vi "Process.vi"(8 "error in":errorcluster, 11 "UI.Lockin.Main":refnum<class "UI.Lockin.lvclass">) -> (0 "error out":errorcluster, 3 "UI.Lockin.Main out":refnum<class "UI.Lockin.lvclass">)   [LabVIEW 2019, in "UI.Lockin.lvclass"]
doc: "---------------------------------------------------------------\nJKI State Machine Objects™\nhttp://jki.net/state-machine-objects/\nCopyright (C) 2005-2015, JKI <info@jki.net>\nALL RIGHTS RESERVED"
uses:
  UI.Lockin.lvclass
  C:/Program Files (x86)/National Instruments/LabVIEW 2019/vi.lib/JKI/JKI SMO/SMO/SMO.lvclass
  <vilib>/JKI/JKI SMO/SMO/SMO.lvclass/SMO.ctl
  <vilib>/JKI/JKI SMO/SMO/Private/ReftoDVR--SMO.vi
  <userlib>/LevyLab/Instrument Framework/SMOs/Instrument UI/Instrument UI.lvclass
  C:/Program Files (x86)/National Instruments/LabVIEW 2019/vi.lib/JKI/JKI SMO/SMO.UI/SMO.UI.lvclass
  <vilib>/JKI/JKI SMO/SMO/SMO.lvclass
  <vilib>/JKI/JKI SMO/SMO.UI/SMO.UI.lvclass
panel:
  in  "configGenerator":bool
  in  "Shutdown":bool
  in  "configDSP":bool
  in  "configDAQ":bool
  in  "show Scope":bool
  # "For instructions on how to use the JKI State Machine Objects, examples and video tutorials, visit:\nhttp://jki.net/state-machine-objects/\n\nJKI State Machine Objects™\nhttp://jki.net/state-machine-objects/\nCopyright (C) 2005-2015, JKI <info@jki.net>\nALL RIGHTS RESERVED"
  # "mainUI"
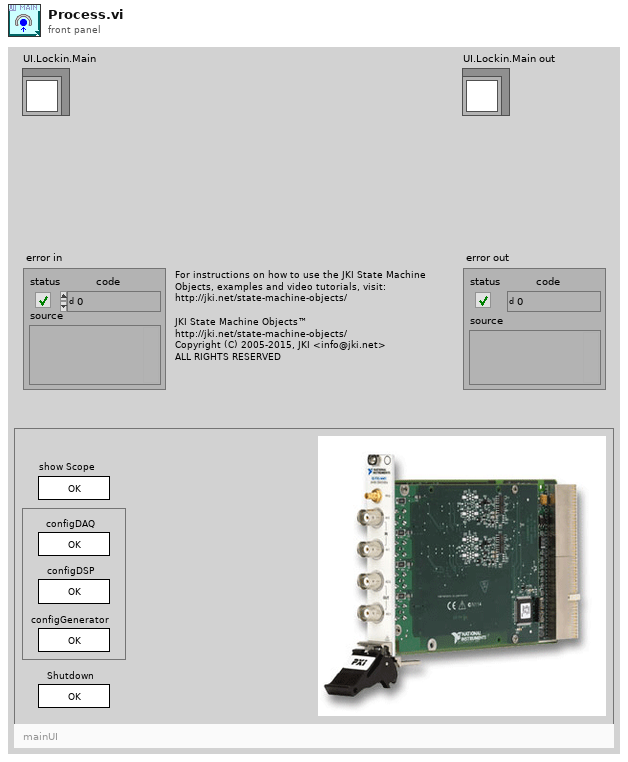
[diagram p1: front panel]
types:
  T1 = enum32{"invalid app kind", "Development System", "Run Time System", "Student Edition", "Embedded LabVIEW", "Evaluation", "Custom"}
  T2 = enum32{"Invalid", "Standard", "Closed", "Hidden", "Minimized", "Maximized"}
  T3 = enum32{"Bad", "Idle", "Run top level", "Running"}
  T4 = cluster{"Core":cluster{"Current VI Reference":refnum<vi>, "Close Panel on Exit?":bool, "error":errorcluster}, "SelfRef":refnum<class "UI.Lockin.lvclass">}
  T5 = cluster{"Current VI Reference":refnum<vi>, "Close Panel on Exit?":bool, "error":errorcluster}
  T6 = typedef "SMO.lvclass/Protected Events.ctl" = cluster{"StopProcesses":refnum<user-event>, "AbortProcesses":refnum<user-event>, "Config Changed":refnum<user-event>, "Dependency":refnum<user-event>}
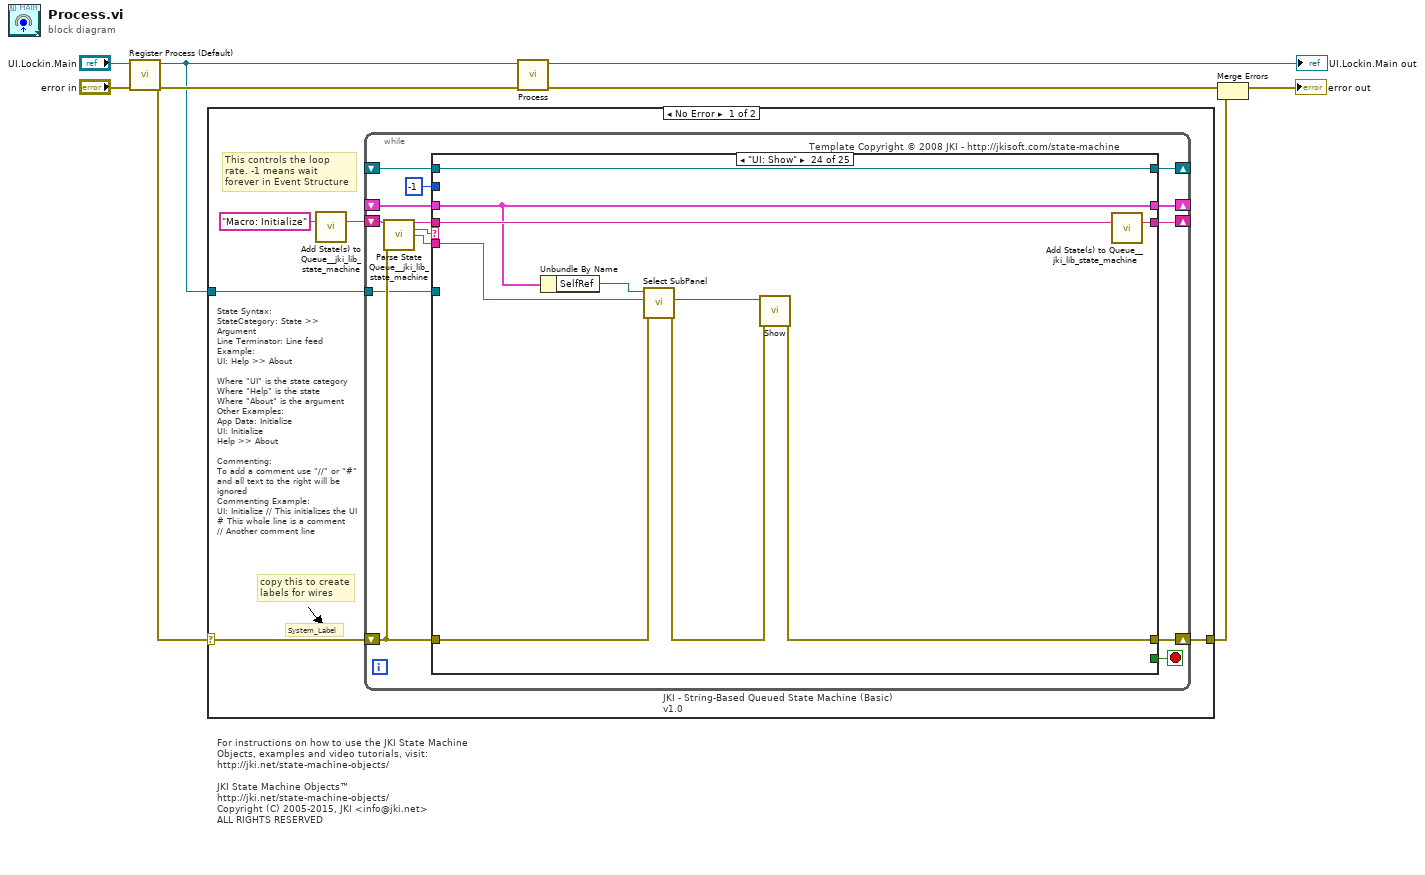
[diagram p0: block diagram]
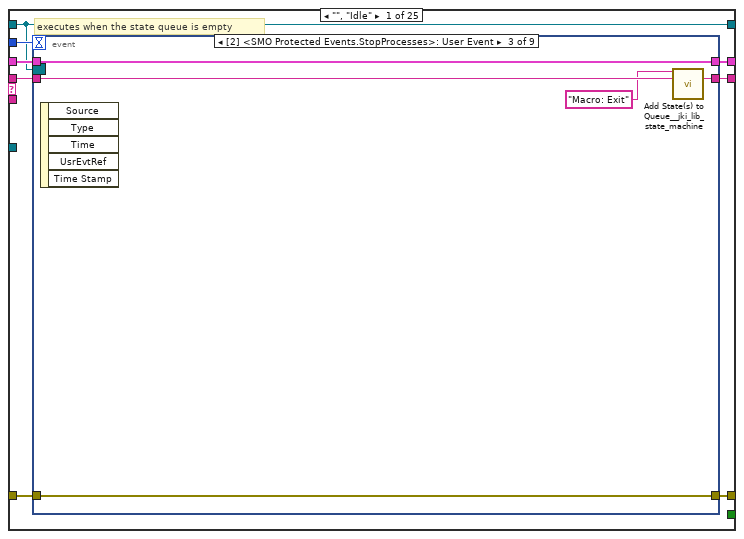
[diagram p2: hidden frame]
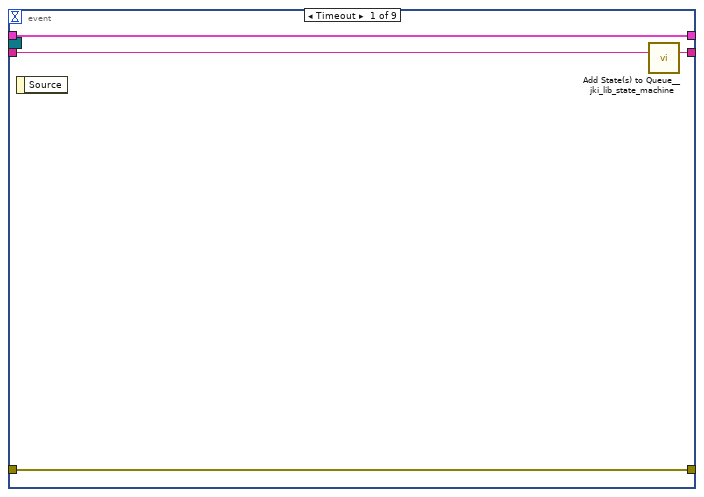
[diagram p3: hidden frame]
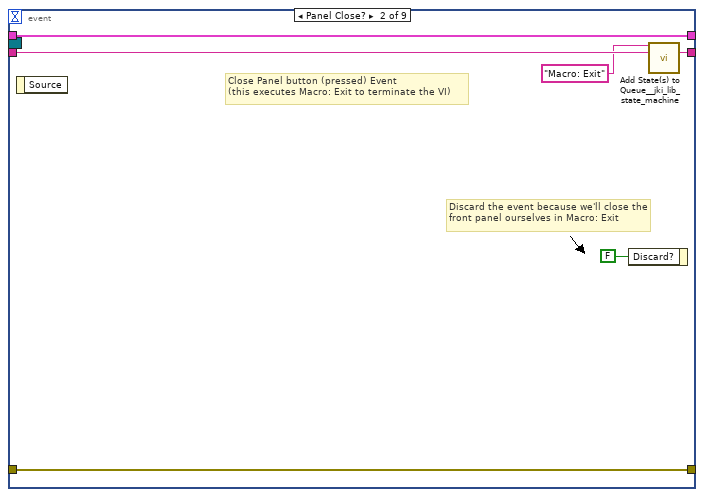
[diagram p4: hidden frame]
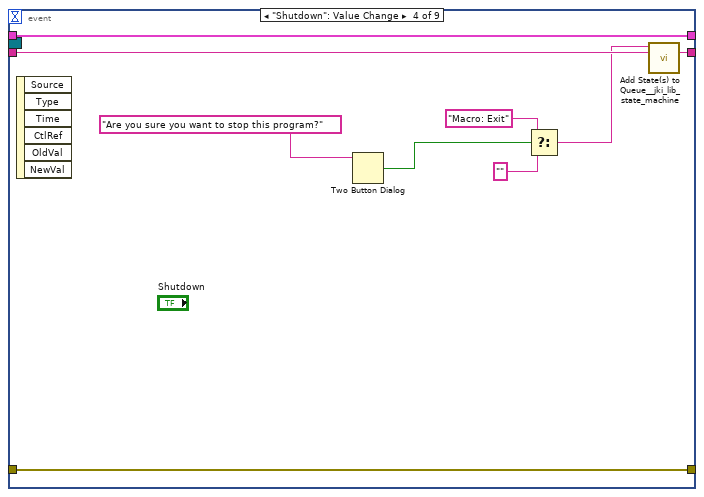
[diagram p5: hidden frame]
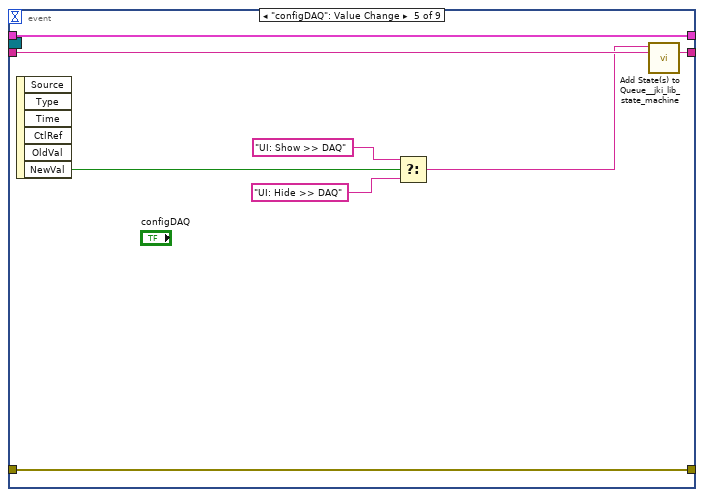
[diagram p6: hidden frame]
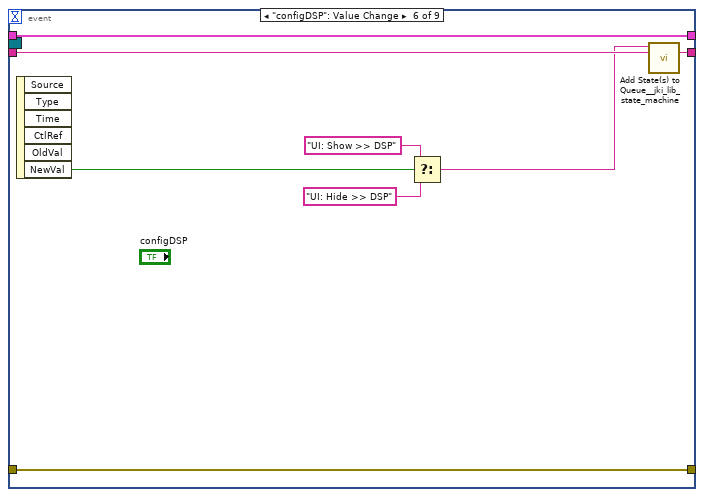
[diagram p7: hidden frame]
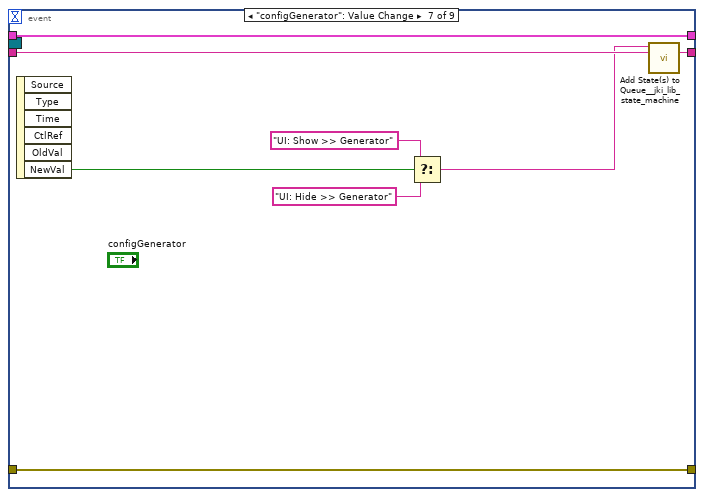
[diagram p8: hidden frame]
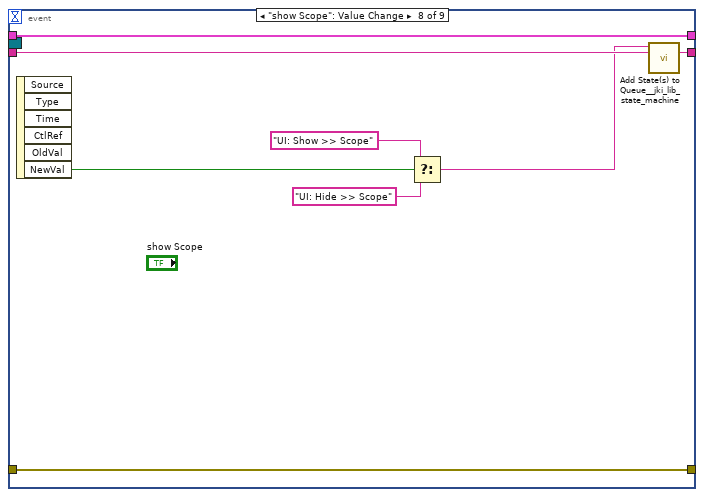
[diagram p9: hidden frame]
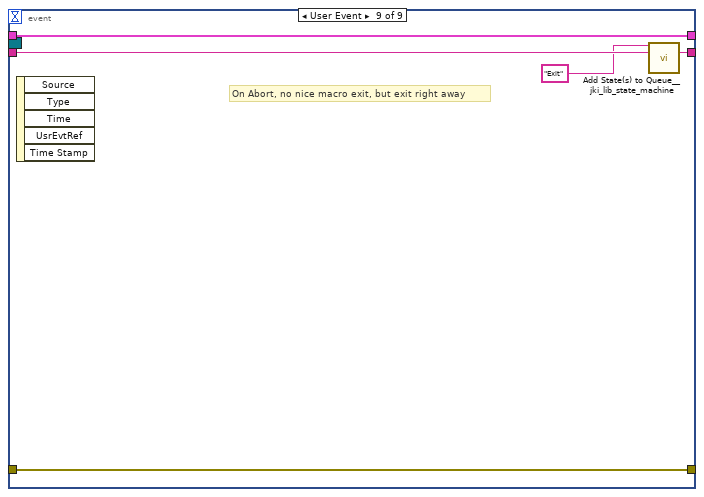
[diagram p10: hidden frame]
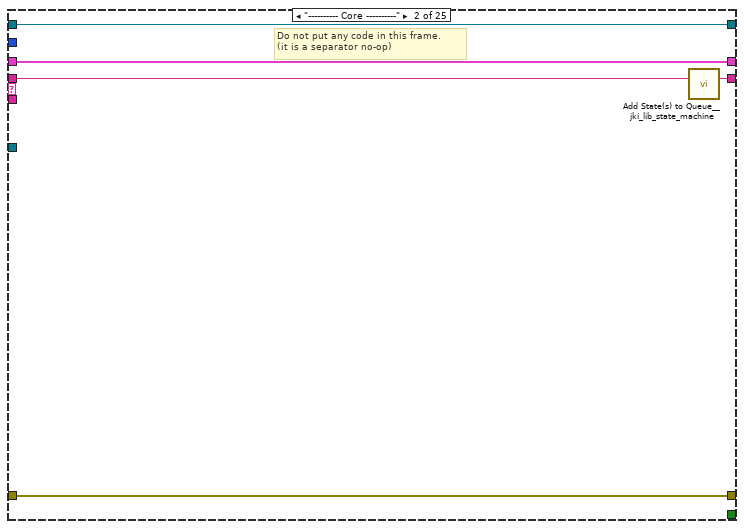
[diagram p11: hidden frame]
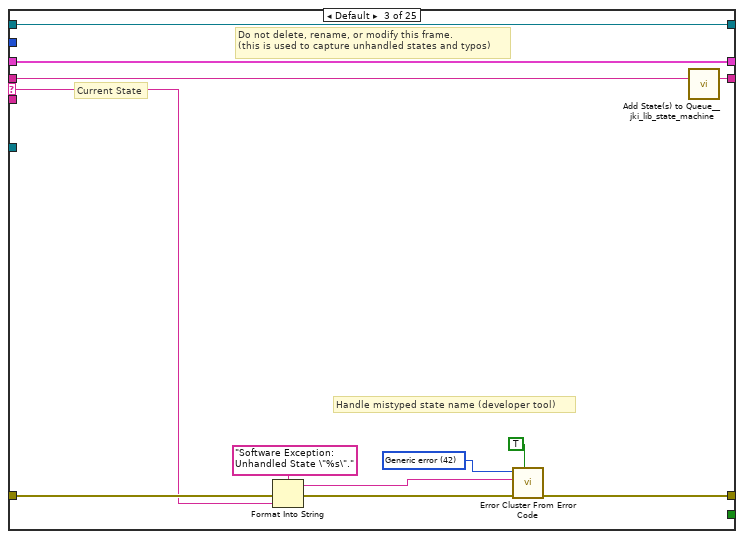
[diagram p12: hidden frame]
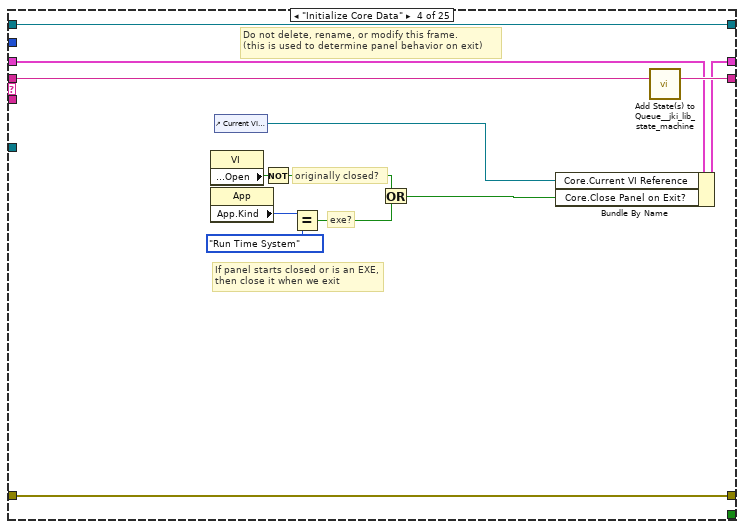
[diagram p13: hidden frame]
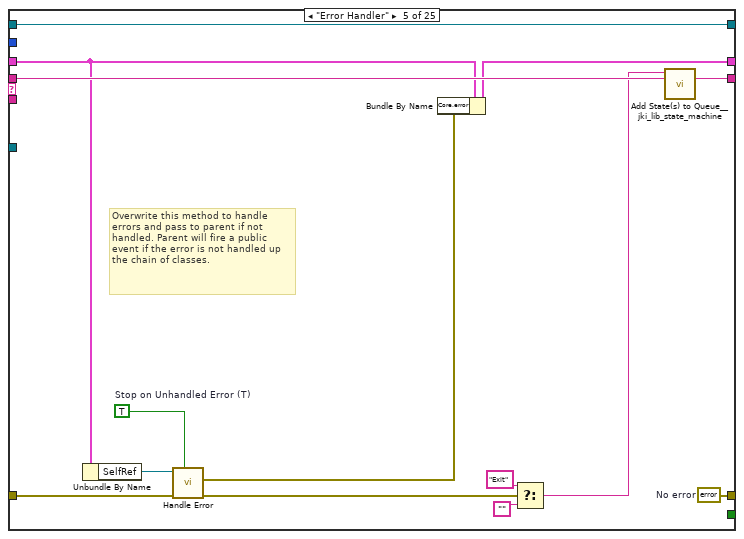
[diagram p14: hidden frame]
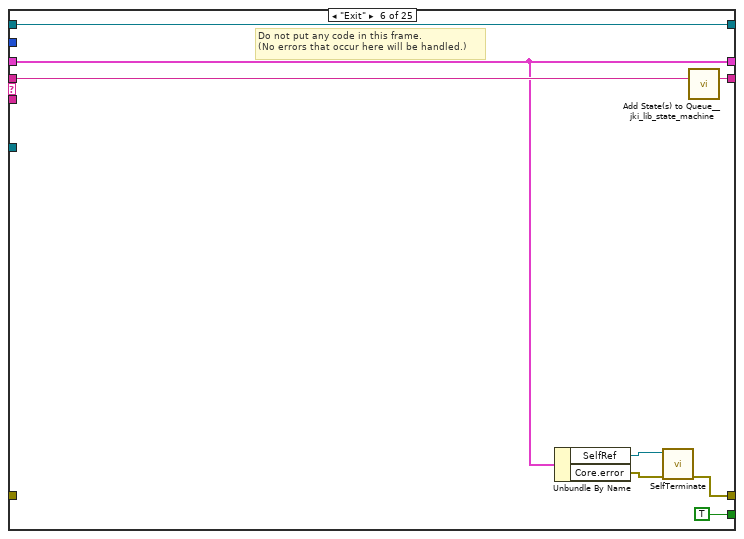
[diagram p15: hidden frame]
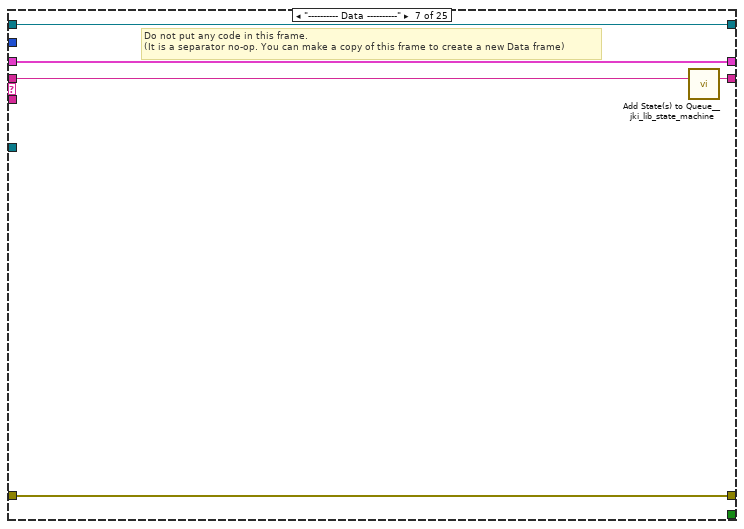
[diagram p16: hidden frame]
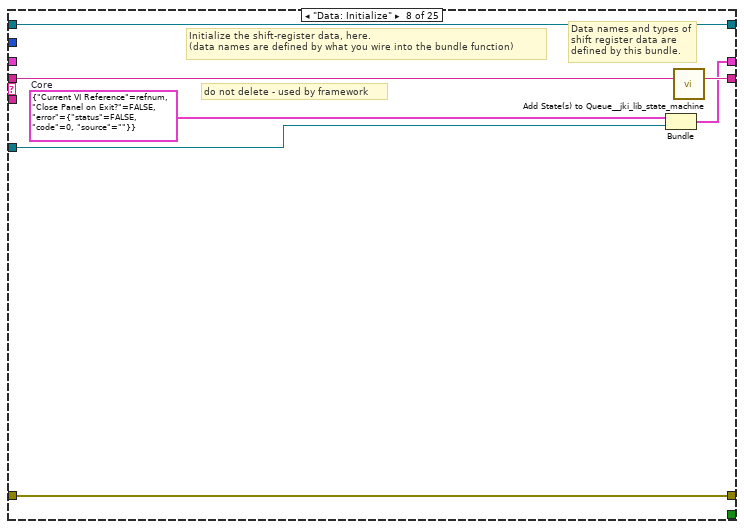
[diagram p17: hidden frame]
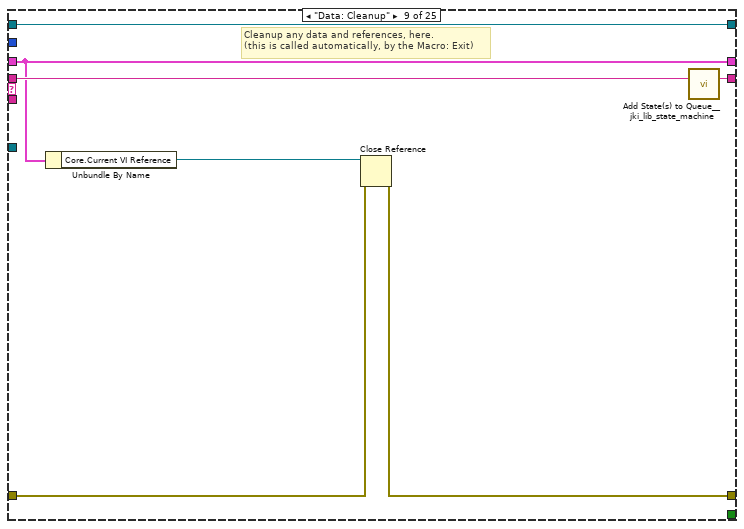
[diagram p18: hidden frame]
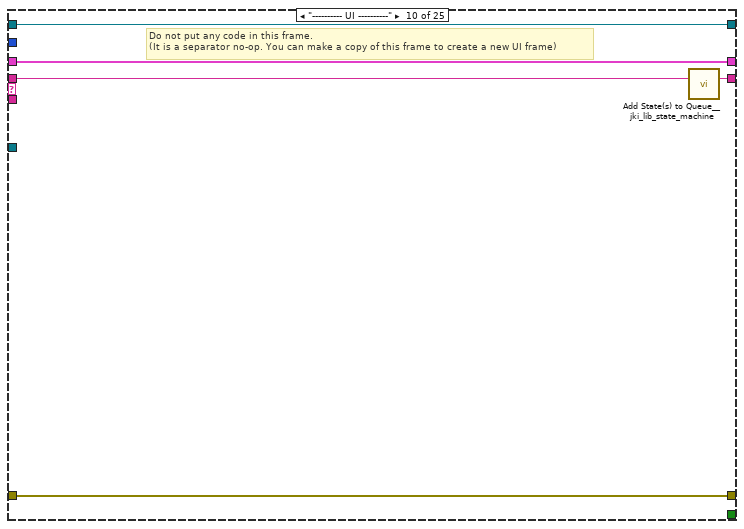
[diagram p19: hidden frame]
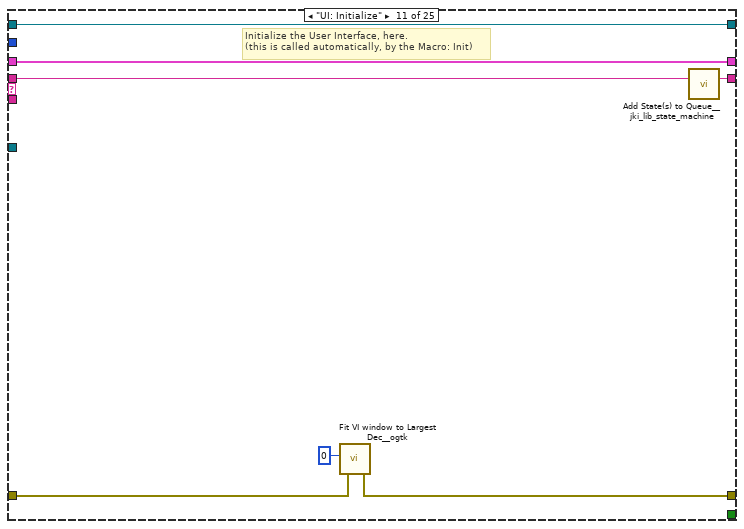
[diagram p20: hidden frame]
diagram:
  # "For instructions on how to use the JKI State Machine Objects, examples and video tutorials, visit:\nhttp://jki.net/state-machine-objects/\n\nJKI State Machine Objects™\nhttp://jki.net/state-machine-objects/\nCopyright (C) 2005-2015, JKI <info@jki.net>\nALL RIGHTS RESERVED"
  n1 = call <vilib>:"Register Process (Default).vi"("error in (no error)"="error in", "SMO"="UI.Lockin.Main") -> ("error out"=w5:errorcluster, "SelfRef"=w4:refnum<class "UI.Lockin.lvclass">)  [unwired: 8 in]
  n2 = case shown="No Error" w5 {
    selector: w5 -> [w10 w332]
    tunnel: w4 -> [w11 _]
    tunnel: [w9 w332] -> w1
    frame No Error {
      # "State Syntax:\nStateCategory: State >> Argument\nLine Terminator: Line feed\nExample:\nUI: Help >> About\n\nWhere \"UI\" is the state category\nWhere \"Help\" is the state\nWhere \"About\" is the argument\nOther Examples:\nApp Data: Initialize\nUI: Initialize\nHelp >> About\n\nCommenting:\nTo add a comment use \"//\" or \"#\" and all text to the right will be ignored\nCommenting Example:\nUI: Initialize // This initializes the UI\n# This whole line is a comment\n// Another comment line"
      # "copy this to create labels for wires"
      # "This controls the loop rate. -1 means wait forever in Event Structure"
      # "System_Label"
      n3 = call <vilib>:"Add State(s) to Queue__jki_lib_state_machine.vi"("State(s) in (\"\")"="Macro: Initialize") -> ("States Out"=w13:string)  [unwired: 14 in]
      n4 = while "JKI - String-Based Queued State Machine (Basic) v1.0" {
        shift-right: [w20] -> _
        shift-left: _ -> [w19]
        shift-right: [w23] -> w9
        shift-left: w10 -> [w17]
        shift-right: [w22] -> _
        shift-left: w13 -> [w24]
        tunnel: w11 -> [w16]
        shift-right: [w15] -> _
        shift-left: _ -> [w14]
        stop <- w21 stop-if-true
        # "Template Copyright © 2008 JKI - http://jkisoft.com/state-machine"
        n5 = call <vilib>:"Parse State Queue__jki_lib_state_machine.vi"("State Queue"=w24, "Error In (no error)"=w17) -> ("Remaining States"=w26:string, "Current State"=w27:string, "Arguments"=w25:string)  [unwired: 11 in]
        n6 = case shown="\"UI: Show\"" w27 {
          selector: w27 -> [_ _ w103 _ _ _ _ _ _ _ _ _ _ _ _ _ _ _ _ _ _ _ _ _ _]
          tunnel: w26 -> [w35 w101 w107 w126 w140 w148 w153 w160 w167 w172 w179 w186 w202 w234 w248 w262 w267 w278 w285 w290 w300 w306 w311 w321 w331]
          tunnel: w25 -> [_ _ _ _ _ _ _ _ _ _ _ w180 w196 _ _ _ _ _ _ _ _ _ _ w316 w327]
          tunnel: w19 -> [w33 w98 w105 w117 w134 w144 w150 _ w162 w169 w177 w184 w198 w231 w244 w249 w264 w275 w282 w287 w298 w304 w309 w318 w322]
          tunnel: [w32 w99 w109 w123 w135 w143 w151 w155 w163 w170 w174 w181 w199 w232 w246 w260 w265 w269 w280 w288 w294 w302 w307 w312 w323] -> w23
          tunnel: w17 -> [w31 w99 w108 w123 w136 _ w151 w155 w164 w170 w173 w182 w200 w232 w246 w260 w265 w270 w279 w288 w291 w302 w307 w315 w325]
          tunnel: [w34 w100 w106 w125 w139 w147 w152 w159 w166 w171 w178 w185 w201 w233 w247 w261 w266 w277 w284 w289 w299 w305 w310 w320 w330] -> w22
          tunnel: [_ _ _ _ _ TRUE _ _ _ _ _ _ _ _ _ _ _ _ _ _ _ _ _ _ _] -> w21
          tunnel: [w30 w98 w105 w124 w133 w144 w150 w158 w162 w169 w177 w184 w198 w231 w244 w249 w264 w275 w282 w287 w298 w304 w309 w318 w322] -> w20
          tunnel: -1 ("Timeout") -> [w29 _ _ _ _ _ _ _ _ _ _ _ _ _ _ _ _ _ _ _ _ _ _ _ _]
          tunnel: w16 -> [_ _ _ _ _ _ _ w154 _ _ _ _ _ _ _ _ _ _ _ _ _ _ _ _ _]
          tunnel: [w28 w97 w102 w114 w138 w145 w149 w157 w161 w168 w176 w183 w195 w230 w245 w254 w263 w276 w283 w286 w297 w303 w308 w319 w329] -> w15
          tunnel: w14 -> [w28 w97 w102 w114 w138 w145 w149 w157 w161 w168 w176 w183 w195 w230 w245 w254 w263 w276 w283 w286 _ w303 w308 w319 w329]
          frame "", "Idle" {
            # "executes when the state queue is empty"
            n7 = event shown="[2] <SMO Protected Events.StopProcesses>: User Event" {
              selector: w28 -> [_ _ _ _ _ _ _ _ _]
              dyn-events: _ -> [_ _ _ _ _ _ _ _ _]
              timeout: w29 -> [_ _ _ _ _ _ _ _ _]
              tunnel: w35 -> [w39 w45 w50 w59 w67 w75 w83 w91 w96]
              tunnel: [w38 w44 w49 w58 w66 w74 w82 w90 w95] -> w34
              tunnel: w33 -> [w37 w42 w47 w56 w64 w72 w80 w88 w93]
              tunnel: [w36 w43 w48 w57 w65 w73 w81 w89 w94] -> w32
              tunnel: w31 -> [w36 w43 w48 w57 w65 w73 w81 w89 w94]
              tunnel: [w37 w42 w47 w56 w64 w72 w80 w88 w93] -> w30
              event Timeout {
                n8 = event-data() -> ()  [unwired: 1 in, 1 out]
                n9 = call <vilib>:"Add State(s) to Queue__jki_lib_state_machine.vi"("State(s) in (\"\")"=w39) -> ("States Out"=w38:string)  [unwired: 14 in]
              }
              event Panel Close? {
                # "Discard the event because we'll close the front panel ourselves in Macro: Exit"
                # "Close Panel button (pressed) Event\n(this executes Macro: Exit to terminate the VI)"
                n10 = event-data() -> ()  [unwired: 1 in, 1 out]
                n11 = event-data("Discard?"=FALSE) -> ()  [unwired: 1 in, 1 out]
                n12 = call <vilib>:"Add State(s) to Queue__jki_lib_state_machine.vi"("State(s) in Front (\"\")"="Macro: Exit", "State(s) in (\"\")"=w45) -> ("States Out"=w44:string)  [unwired: 13 in]
              }
              event User Event {
                n13 = event-data() -> ()  [unwired: 1 in, 5 out]
                n14 = call <vilib>:"Add State(s) to Queue__jki_lib_state_machine.vi"("State(s) in Front (\"\")"="Macro: Exit", "State(s) in (\"\")"=w50) -> ("States Out"=w49:string)  [unwired: 13 in]
              }
              event "Shutdown": Value Change {
                n15 = event-data() -> ()  [unwired: 1 in, 6 out]
                n16 = Two Button Dialog(message="Are you sure you want to stop this program?") -> (T button?=w55:bool)  [unwired: 2 in]
                n17 = Select(t="Macro: Exit", s=w55, f="") -> (s? t:f=w51:string)
                n18 = call <vilib>:"Add State(s) to Queue__jki_lib_state_machine.vi"("State(s) in Front (\"\")"=w51, "State(s) in (\"\")"=w59) -> ("States Out"=w58:string)  [unwired: 13 in]
              }
              event "configDAQ": Value Change {
                n19 = event-data() -> ("NewVal"=w63:bool)  [unwired: 1 in, 5 out]
                n20 = Select(t="UI: Show >> DAQ", s=w63, f="UI: Hide >> DAQ") -> (s? t:f=w60:string)
                n21 = call <vilib>:"Add State(s) to Queue__jki_lib_state_machine.vi"("State(s) in Front (\"\")"=w60, "State(s) in (\"\")"=w67) -> ("States Out"=w66:string)  [unwired: 13 in]
              }
              event "configDSP": Value Change {
                n22 = event-data() -> ("NewVal"=w71:bool)  [unwired: 1 in, 5 out]
                n23 = Select(t="UI: Show >> DSP", s=w71, f="UI: Hide >> DSP") -> (s? t:f=w70:string)
                n24 = call <vilib>:"Add State(s) to Queue__jki_lib_state_machine.vi"("State(s) in Front (\"\")"=w70, "State(s) in (\"\")"=w75) -> ("States Out"=w74:string)  [unwired: 13 in]
              }
              event "configGenerator": Value Change {
                n25 = event-data() -> ("NewVal"=w79:bool)  [unwired: 1 in, 5 out]
                n26 = Select(t="UI: Show >> Generator", s=w79, f="UI: Hide >> Generator") -> (s? t:f=w78:string)
                n27 = call <vilib>:"Add State(s) to Queue__jki_lib_state_machine.vi"("State(s) in Front (\"\")"=w78, "State(s) in (\"\")"=w83) -> ("States Out"=w82:string)  [unwired: 13 in]
              }
              event "show Scope": Value Change {
                n28 = event-data() -> ("NewVal"=w87:bool)  [unwired: 1 in, 5 out]
                n29 = Select(t="UI: Show >> Scope", s=w87, f="UI: Hide >> Scope") -> (s? t:f=w86:string)
                n30 = call <vilib>:"Add State(s) to Queue__jki_lib_state_machine.vi"("State(s) in Front (\"\")"=w86, "State(s) in (\"\")"=w91) -> ("States Out"=w90:string)  [unwired: 13 in]
              }
              event User Event {
                # "On Abort, no nice macro exit, but exit right away"
                n31 = event-data() -> ()  [unwired: 1 in, 5 out]
                n32 = call <vilib>:"Add State(s) to Queue__jki_lib_state_machine.vi"("State(s) in Front (\"\")"="Exit", "State(s) in (\"\")"=w96) -> ("States Out"=w95:string)  [unwired: 13 in]
              }
            }
          }
          frame "---------- Core ----------" {
            # "Do not put any code in this frame.\n(it is a separator no-op)"
            n33 = call <vilib>:"Add State(s) to Queue__jki_lib_state_machine.vi"("State(s) in (\"\")"=w101) -> ("States Out"=w100:string)  [unwired: 14 in]
          }
          frame Default {
            w112 = 42 items=["No error", "Argument error", "Memory is full", "Out of zone", "End of file", "File already open", "Generic file I/O error", "File not found", "File permission error", "Disk is full", "Duplicate path", "Too many files open", "System feature not enabled", "Resource file not found", "Cannot add resource", "Resource not found", "Image not found", "Image memory error", "Pen does not exist", "Config type invalid", "Config token not found", "Config parse error", "Config memory error", "Bad external code format", "Bad external code offset", "External code not present", "Null window", "Destroy window error", "Null menu", "Print aborted", "Bad print record", "Print driver error", "Windows error during printing", "Memory error during printing", "Print dialog error", "Generic print error", "Invalid device refnum", "Device not found", "Device parameter error", "Device unit error", "Cannot open device", "Device call aborted", "Generic error", "Cancelled by user", "Object ID too low", "Object ID too high", "Object not in heap", "Unknown heap", "Unknown object (invalid DefProc)", "Unknown object (DefProc not in table)", "Message out of range", "Invalid (null) method", "Unknown message", "Manager call not supported", "Bad address", "Network operation in progress", "Network operation timed out", "Connection is busy", "Network attribute not supported", "Network error", "Address in use", "System out of memory", "Connection aborted", "Connection refused", "Not connected", "Already connected", "Connection closed", "Initialization error (interapplication manager)", "Bad occurrence", "Wait on unbound occurrence handler", "Occurrence queue overflow", "Datalog type conflict", "Unused", "Unrecognized type (interapplication manager)", "Memory corrupt", "Failed to make temporary DLL", "Old CIN version", "Drag socket not found", "Failed to load drop-object", "Failed to register OLE object", "Failed to release OLE object", "Format specifier type mismatch", "Unknown format specifier", "Too few format specifiers", "Too many format specifiers", "Scan failed", "Newer CIN version", "Error converting to variant", "Runtime menu error", "Password tampered", "Variant attribute not found", "Incompatible variant data type", "Event data is not available", "Event Store is not present", "Occurrence is not found", "Event Queue is not created", "Event info is not available", "Refnum passed is NULL", "Error retrieving Class GUID", "Error retrieving CoClass GUID", "Error retrieving TypeLib GUID.", "Bad built application magic bytes.", "Specific driver is different from the specific driver associated with the Logical Name.", "There is no session opened to the class driver.", "Max Error", "MAX - Error with config objects", "MAX - Error loading configuration", "MAX - Group not supported"]
            # "Current State"
            # "Do not delete, rename, or modify this frame.\n(this is used to capture unhandled states and typos)"
            # "Handle mistyped state name (developer tool)"
            n34 = Format Into String(format string="Software Exception: Unhandled State \"%s\"." ("message"), error in=w108, w103) -> (resulting string=w111:string, error out=w110:errorcluster)  [unwired: 1 in]
            n35 = call <vilib>:"Error Cluster From Error Code.vi"("show call chain? (False)"=TRUE, "error in (no error)"=w110, "error message (\"\")"=w111, "error code (0)"=w112) -> ("error out"=w109:errorcluster)  [unwired: 5 in]
            n36 = call <vilib>:"Add State(s) to Queue__jki_lib_state_machine.vi"("State(s) in (\"\")"=w107) -> ("States Out"=w106:string)  [unwired: 14 in]
          }
          frame "Initialize Core Data" {
            # "Do not delete, rename, or modify this frame.\n(this is used to determine panel behavior on exit)"
            # "originally closed?"
            # "exe?"
            # "If panel starts closed or is an EXE, then close it when we exit"
            n37 = property class="VI"() -> ("Front Panel.Open"=w122:bool)  [unwired: 2 in, 2 out]
            n38 = property class="App"() -> ("App.Kind"=w121:T1)  [unwired: 2 in, 2 out]
            n39 = control-ref of="Current VI Reference"() -> (w115:refnum<vi>)
            n40 = Not(x=w122) -> (.not. x?=w119:bool)
            n41 = Equal?(x=w121, y=T1."Run Time System" ("Application:Kind")) -> (x = y?=w118:bool)
            n42 = Or(x=w119, y=w118) -> (x .or. y?=w116:bool)
            n43 = Bundle By Name(cluster=w117, "Core.Current VI Reference"=w115, "Core.Close Panel on Exit?"=w116) -> (w124:T4)
            n44 = call <vilib>:"Add State(s) to Queue__jki_lib_state_machine.vi"("State(s) in (\"\")"=w126) -> ("States Out"=w125:string)  [unwired: 14 in]
          }
          frame "Error Handler" {
            w127 = TRUE  # Stop on Unhandled Error (T)
            w135 = errorcluster {"status"=FALSE, "code"=0, "source"=""}  # No error
            # "Overwrite this method to handle errors and pass to parent if not handled. Parent will fire a public event if the error is not handled up the chain of classes."
            n45 = Unbundle By Name(w134) -> ("SelfRef"=w137:refnum<class "UI.Lockin.lvclass">)
            n46 = call-dynamic "Handle Error.vi"("Stop on Unhandled Error (T)"=w127, "error in"=w136, "SMO"=w137) -> ("handling error"=w128:errorcluster, "Unhandled error"=w131:errorcluster)  [unwired: 6 in, 1 out]
            n47 = Bundle By Name(cluster=w134, "Core.error"=w131) -> (w133:T4)
            n48 = Select(t="Exit", s=w128, f="") -> (s? t:f=w132:string)
            n49 = call <vilib>:"Add State(s) to Queue__jki_lib_state_machine.vi"("State(s) in Front (\"\")"=w132, "State(s) in (\"\")"=w140) -> ("States Out"=w139:string)  [unwired: 13 in]
          }
          frame "Exit" {
            # "Do not put any code in this frame.\n(No errors that occur here will be handled.)"
            n50 = Unbundle By Name(w144) -> ("SelfRef"=w142:refnum<class "UI.Lockin.lvclass">, "Core.error"=w141:errorcluster)
            n51 = call <vilib>:"SelfTerminate.vi"("error in (no error)"=w141, "SMO in"=w142) -> ("error out"=w143:errorcluster)  [unwired: 8 in, 1 out]
            n52 = call <vilib>:"Add State(s) to Queue__jki_lib_state_machine.vi"("State(s) in (\"\")"=w148) -> ("States Out"=w147:string)  [unwired: 14 in]
          }
          frame "---------- Data ----------" {
            # "Do not put any code in this frame.\n(It is a separator no-op. You can make a copy of this frame to create a new Data frame)"
            n53 = call <vilib>:"Add State(s) to Queue__jki_lib_state_machine.vi"("State(s) in (\"\")"=w153) -> ("States Out"=w152:string)  [unwired: 14 in]
          }
          frame "Data: Initialize" {
            w156 = T5 {"Current VI Reference"=refnum, "Close Panel on Exit?"=FALSE, "error"={"status"=FALSE, "code"=0, "source"=""}}  # Core
            # "do not delete - used by framework"
            # "Data names and types of shift register data are defined by this bundle."
            # "Initialize the shift-register data, here.\n(data names are defined by what you wire into the bundle function)"
            n54 = Bundle("Core"=w156, "SelfRef"=w154) -> (w158:T4)  [unwired: 1 in]
            n55 = call <vilib>:"Add State(s) to Queue__jki_lib_state_machine.vi"("State(s) in (\"\")"=w160) -> ("States Out"=w159:string)  [unwired: 14 in]
          }
          frame "Data: Cleanup" {
            # "Cleanup any data and references, here.\n(this is called automatically, by the Macro: Exit)"
            n56 = Unbundle By Name(w162) -> ("Core.Current VI Reference"=w165:refnum<vi>)
            n57 = Close Reference(reference=w165, error in (no error)=w164) -> (error out=w163:errorcluster)
            n58 = call <vilib>:"Add State(s) to Queue__jki_lib_state_machine.vi"("State(s) in (\"\")"=w167) -> ("States Out"=w166:string)  [unwired: 14 in]
          }
          frame "---------- UI ----------" {
            # "Do not put any code in this frame.\n(It is a separator no-op. You can make a copy of this frame to create a new UI frame)"
            n59 = call <vilib>:"Add State(s) to Queue__jki_lib_state_machine.vi"("State(s) in (\"\")"=w172) -> ("States Out"=w171:string)  [unwired: 14 in]
          }
          frame "UI: Initialize" {
            # "Initialize the User Interface, here.\n(this is called automatically, by the Macro: Init)"
            n60 = call <userlib>:"Fit VI window to Largest Dec__ogtk.vi"("error in (no error)"=w173, "border spacing (2 px)"=0) -> ("error out"=w174:errorcluster)  [unwired: 4 in, 1 out]
            n61 = call <vilib>:"Add State(s) to Queue__jki_lib_state_machine.vi"("State(s) in (\"\")"=w179) -> ("States Out"=w178:string)  [unwired: 14 in]
          }
          frame "UI: Cursor Set" {
            # "Argument"
            # "Initialize the User Interface, here.\n(this is called automatically, by the Macro: Init)"
            n62 = disable-structure shown="Default" {
              disable-tunnel: w182 -> [w187 w190]
              disable-tunnel: [w187 w189] -> w181
              disable-tunnel: w180 -> [_ w188]
              frame condition #0 {
              }
              frame condition #1 (active) {
                n63 = case shown="\"Idle\", Default" w188 {
                  tunnel: w190 -> [w192 w194]
                  tunnel: [w191 w193] -> w189
                  frame "Idle", Default {
                    n64 = call <vilib>:"Unset Busy.vi"("error in (no error)"=w192) -> ("error out"=w191:errorcluster)  [unwired: 10 in]
                  }
                  frame "Busy" {
                    n65 = call <vilib>:"Set Busy.vi"("error in (no error)"=w194) -> ("error out"=w193:errorcluster)  [unwired: 9 in, 1 out]
                  }
                }
              }
            }
            n66 = call <vilib>:"Add State(s) to Queue__jki_lib_state_machine.vi"("State(s) in (\"\")"=w186) -> ("States Out"=w185:string)  [unwired: 14 in]
          }
          frame "UI: Front Panel State" {
            # "Argument"
            # "Set Front Panel Open or Closed\n(Usage: \"UI: Front Panel State >> Open|Close\")"
            n67 = Unbundle By Name(w198) -> ("Core.Current VI Reference"=w197:refnum<vi>)
            n68 = disable-structure shown="Default" {
              disable-tunnel: w200 -> [w206 w229]
              disable-tunnel: [w205 w229] -> w199
              disable-tunnel: w197 -> [w204 _]
              disable-tunnel: w196 -> [w203 _]
              frame condition #0 (active) {
                n69 = case shown="\"Close\"" w203 {
                  tunnel: w206 -> [w210 w223]
                  tunnel: [w212 w224] -> w205
                  tunnel: w204 -> [w211 w221]
                  frame "Open", Default {
                    n70 = property class="VI"(reference=w211, error in=w210) -> (reference out=w208:refnum<vi>, error out=w209:errorcluster, "FP.State"=w207:T2)
                    n71 = case shown="\"Closed\"" w207 {
                      tunnel: [w215 w218] -> w212
                      tunnel: w209 -> [w214 w218]
                      tunnel: w208 -> [w213 _]
                      frame "Closed" {
                        n72 = invoke class="VI" method="FP.Open"(reference=w213, error in=w214, "Activate"=TRUE, "State"=T2."Standard") -> (error out=w215:errorcluster)  [unwired: 1 in, 4 out]
                      }
                      frame Default {
                      }
                    }
                  }
                  frame "Close" {
                    n73 = property class="VI"(reference=w221, error in=w223) -> (reference out=w220:refnum<vi>, error out=w222:errorcluster, "FP.State"=w219:T2)
                    n74 = case shown="Default" w219 {
                      tunnel: [w225 w228] -> w224
                      tunnel: w222 -> [w225 w227]
                      tunnel: w220 -> [_ w226]
                      frame "Invalid", "Closed" {
                      }
                      frame Default {
                        n75 = invoke class="VI" method="FP.Close"(reference=w226, error in=w227) -> (error out=w228:errorcluster)  [unwired: 1 in, 2 out]
                      }
                    }
                  }
                }
              }
              frame condition #1 {
              }
            }
            n76 = call <vilib>:"Add State(s) to Queue__jki_lib_state_machine.vi"("State(s) in (\"\")"=w202) -> ("States Out"=w201:string)  [unwired: 14 in]
          }
          frame "---------- Macro ----------" {
            # "Do not put any code in this frame.\n(It is a separator no-op. You can make a copy of this frame to create a new Macro frame)"
            n77 = call <vilib>:"Add State(s) to Queue__jki_lib_state_machine.vi"("State(s) in (\"\")"=w234) -> ("States Out"=w233:string)  [unwired: 14 in]
          }
          frame "Macro: Initialize" {
            w239 = "UI: Initialize\n//UI: Front Panel State >> Open"  # UI: Initialize //UI: Front Panel State >> Open
            w235 = "Process: Sync"
            # "Initialization Macro\n(This is called once, when the VI starts)"
            n78 = control-ref of="This VI"() -> (w237:refnum<vi>)
            n79 = property class="VI"(reference=w237) -> ("Exec.State"=w236:T3)  [unwired: 1 in, 2 out]
            n80 = Equal?(x=w236, y=T3."Run top level") -> (x = y?=w242:bool)
            n81 = Select(t=w235, s=w242, f="") -> ()  [unwired: 1 out]
            n82 = call <vilib>:"Add State(s) to Queue__jki_lib_state_machine.vi"("State(s) in Front (\"\")"="Data: Initialize\nInitialize Core Data\nEvents: Register", "State(s) in (\"\")"=w235, "State(s) at Back (\"\")"=w239) -> ("States Out"=w238:string)  [unwired: 12 in]
            n83 = call <vilib>:"Add State(s) to Queue__jki_lib_state_machine.vi"("State(s) in Front (\"\")"=w238, "State(s) in (\"\")"=w248) -> ("States Out"=w247:string)  [unwired: 13 in]
          }
          frame "Macro: Exit" {
            # "Exit Macro\n(This is called once, when the VI exits)"
            n84 = Unbundle By Name(w249) -> ("Core.Close Panel on Exit?"=w259:bool)
            n85 = Select(t="UI: Front Panel State >> Close", s=w259, f="") -> (s? t:f=w256:string)
            n86 = call <vilib>:"Add State(s) to Queue__jki_lib_state_machine.vi"("State(s) in Front (\"\")"="Data: Cleanup\nEvents: Unregister\nProcess: SelfTerminate", "State(s) in (\"\")"="Process: Sync", "State(s) at Back (\"\")"="Exit") -> ("States Out"=w251:string)  [unwired: 12 in]
            n87 = call <vilib>:"Add State(s) to Queue__jki_lib_state_machine.vi"("State(s) in (\"\")"=w256, "State(s) at Back (\"\")"=w251) -> ("States Out"=w255:string)  [unwired: 13 in]
            n88 = call <vilib>:"Add State(s) to Queue__jki_lib_state_machine.vi"("State(s) in Front (\"\")"=w255, "State(s) in (\"\")"=w262) -> ("States Out"=w261:string)  [unwired: 13 in]
          }
          frame "---------- Process ----------" {
            # "Template Separator\n(You can make a copy of, or modify, this frame)"
            n89 = call <vilib>:"Add State(s) to Queue__jki_lib_state_machine.vi"("State(s) in (\"\")"=w267) -> ("States Out"=w266:string)  [unwired: 14 in]
          }
          frame "Process: Sync" {
            n90 = Unbundle By Name(w275) -> ("SelfRef"=w271:refnum<class "UI.Lockin.lvclass">)
            n91 = call <vilib>:"WaitOnProcessSync.vi"("error in (no error)"=w270, "SMO"=w271) -> ("error out"=w269:errorcluster, "Don't run?"=w274:bool)  [unwired: 7 in, 1 out]
            n92 = Select(t="Data: Cleanup\nEvents: Unregister\nExit", s=w274, f="") -> (s? t:f=w268:string)
            n93 = call <vilib>:"Add State(s) to Queue__jki_lib_state_machine.vi"("State(s) in Front (\"\")"=w268, "State(s) in (\"\")"=w278) -> ("States Out"=w277:string)  [unwired: 13 in]
          }
          frame "Process: SelfTerminate" {
            # "Template Separator\n(You can make a copy of, or modify, this frame)"
            n94 = Unbundle By Name(w282) -> ("SelfRef"=w281:refnum<class "UI.Lockin.lvclass">)
            n95 = call <vilib>:"SelfTerminate.vi"("error in (no error)"=w279, "SMO in"=w281) -> ("error out"=w280:errorcluster)  [unwired: 8 in, 1 out]
            n96 = call <vilib>:"Add State(s) to Queue__jki_lib_state_machine.vi"("State(s) in (\"\")"=w285) -> ("States Out"=w284:string)  [unwired: 14 in]
          }
          frame "---------- Events ----------" {
            # "Template Separator\n(You can make a copy of, or modify, this frame)"
            n97 = call <vilib>:"Add State(s) to Queue__jki_lib_state_machine.vi"("State(s) in (\"\")"=w290) -> ("States Out"=w289:string)  [unwired: 14 in]
          }
          frame "Events: Register" {
            # "Expand to add\nmore events"
            n98 = Unbundle By Name(w298) -> ("SelfRef"=w295:refnum<class "UI.Lockin.lvclass">)
            n99 = call <vilib>:"GetProtectedEvents.vi"("SMO"=w295) -> ("error out"=w292:errorcluster, "SMO Protected Events"=w296:T6)  [unwired: 8 in, 1 out]
            n100 = register-events(w296) -> (reference out=w297:refnum<event-registration>, error out=w293:errorcluster)  [unwired: 2 in]
            n101 = Merge Errors(w293, w292, w291) -> (w294:errorcluster)
            n102 = call <vilib>:"Add State(s) to Queue__jki_lib_state_machine.vi"("State(s) in (\"\")"=w300) -> ("States Out"=w299:string)  [unwired: 14 in]
          }
          frame "Events: Unregister" {
            n103 = Unregister For Events(event registration refnum=w303, error in=w302) -> (error out=w301:errorcluster)
            n104 = call <vilib>:"Clear Errors.vi"("error in (no error)"=w301) -> ()  [unwired: 5 in, 2 out]
            n105 = call <vilib>:"Add State(s) to Queue__jki_lib_state_machine.vi"("State(s) in (\"\")"=w306) -> ("States Out"=w305:string)  [unwired: 14 in]
          }
          frame "---------- Action ----------" {
            n106 = call <vilib>:"Add State(s) to Queue__jki_lib_state_machine.vi"("State(s) in (\"\")"=w311) -> ("States Out"=w310:string)  [unwired: 14 in]
          }
          frame "UI: Show" {
            n107 = Unbundle By Name(w318) -> ("SelfRef"=w317:refnum<class "UI.Lockin.lvclass">)
            n108 = call "Select SubPanel.vi"("error in (no error)"=w315, "Arguments"=w316, "UI.Lockin"=w317) -> ("error out"=w313:errorcluster, "UI_"=w314:refnum<class "Instrument UI.lvclass">)  [unwired: 6 in, 1 out]
            n109 = call <vilib>:"Show.vi"("error in (no error)"=w313, "SMO.UI"=w314) -> ("error out"=w312:errorcluster)  [unwired: 8 in, 1 out]
            n110 = call <vilib>:"Add State(s) to Queue__jki_lib_state_machine.vi"("State(s) in (\"\")"=w321) -> ("States Out"=w320:string)  [unwired: 14 in]
          }
          frame "UI: Hide" {
            n111 = Unbundle By Name(w322) -> ("SelfRef"=w328:refnum<class "UI.Lockin.lvclass">)
            n112 = call "Select SubPanel.vi"("error in (no error)"=w325, "Arguments"=w327, "UI.Lockin"=w328) -> ("error out"=w324:errorcluster, "UI_"=w326:refnum<class "Instrument UI.lvclass">)  [unwired: 6 in, 1 out]
            n113 = call <vilib>:"Hide.vi"("error in (no error)"=w324, "SMO.UI"=w326) -> ("error out"=w323:errorcluster)  [unwired: 8 in, 1 out]
            n114 = call <vilib>:"Add State(s) to Queue__jki_lib_state_machine.vi"("State(s) in (\"\")"=w331) -> ("States Out"=w330:string)  [unwired: 14 in]
          }
        }
      }
    }
    frame Error {
    }
  }
  n115 = call-parent "Process.vi"("error in"=w5, "Instrument UI in"=w4) -> ("error out"=w2:errorcluster, "Instrument UI out"=→"UI.Lockin.Main out":refnum<class "UI.Lockin.lvclass">)  [unwired: 8 in]
  n116 = Merge Errors(w2, w1) -> (→"error out":errorcluster)
